vi "missing_Peak2.vi"(8 "Width":dbl=0.02 format="%#_13g", 9 "Average Spacing":dbl=1.0 format="%#_13g") -> (0 "Missing Peaks":i32[](array[numeric])=[3, 4, 7, 8, 9], 3 "Padded Peak Locations":i32[](array[numeric])=[1, 2, 3, 4, 5, 6, 7, 8, 9, 10])   [LabVIEW 2016]
panel:
  in  "array":i32[](array[numeric])
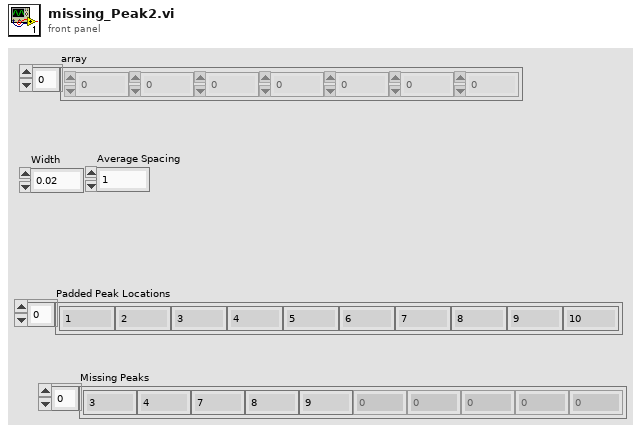
[diagram p1: front panel]
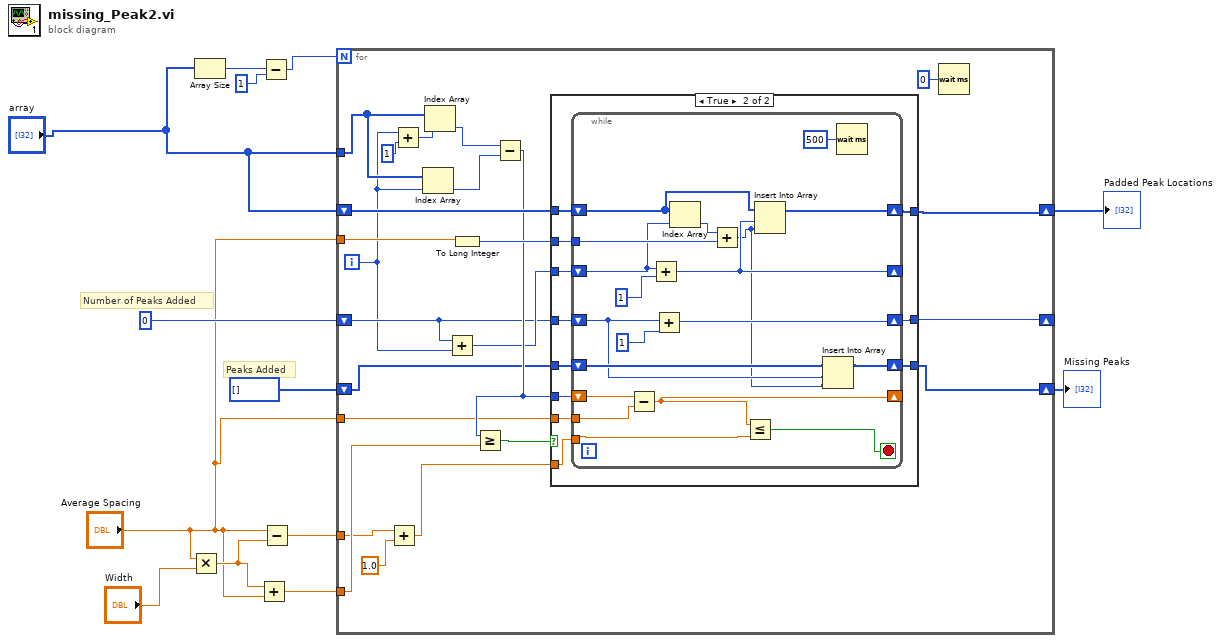
[diagram p0: block diagram]
diagram:
  # "Peaks Added"
  # "Number of Peaks Added"
  n1 = Multiply(x="Average Spacing", y="Width") -> (x*y=w10:dbl)
  n2 = Array Size(array="array") -> (size(s)=w13:i32)
  n3 = Add(x=w10, y="Average Spacing") -> (x+y=w7:dbl)
  n4 = Subtract(x=w13, y=1) -> (x-y=w11:i32)
  n5 = Subtract(x="Average Spacing", y=w10) -> (x-y=w8:dbl)
  n6 = for {
    N: w11 -> [_]
    tunnel: "array" -> [w31]
    tunnel: w8 -> [w19]
    tunnel: w7 -> [w25]
    shift-right: [w29] -> w6
    shift-left: "array" -> [w30]
    tunnel: "Average Spacing" -> [w24]
    shift-right: [w22] -> _
    shift-left: 0 -> [w21]
    shift-right: [w15] -> w3
    shift-left: i32[] [] ("array") -> [w16]
    tunnel: "Average Spacing" -> [w14]
    i -> [w20]
    n7 = Add(x=w19, y=1.0) -> (x+y=w17:dbl)
    n8 = Add(x=w20, y=1) -> (x+y=w36:i32)
    n9 = Index Array(array=w31, index=w20) -> (element=w33:i32)
    n10 = Index Array(array=w31, index=w36) -> (element=w34:i32)
    n11 = Add(x=w21, y=w20) -> (x+y=w23:i32)
    n12 = To Long Integer(number=w24) -> (32bit integer=w28:i32)
    n13 = Subtract(x=w34, y=w33) -> (x-y=w26:i32)
    n14 = Greater Or Equal?(x=w26, y=w25) -> (x >= y?=w32:bool)
    n15 = case shown="True" w32 {
      tunnel: w30 -> [w39 w49]
      tunnel: w26 -> [_ w50]
      tunnel: w23 -> [_ w48]
      tunnel: w28 -> [_ w47]
      tunnel: [w39 w46] -> w29
      tunnel: w21 -> [w38 w45]
      tunnel: [w38 w44] -> w22
      tunnel: w17 -> [_ w43]
      tunnel: w16 -> [w37 w42]
      tunnel: [w37 w41] -> w15
      tunnel: w14 -> [_ w40]
      frame False {
      }
      frame True {
        n16 = while {
          shift-right: [w67] -> _
          shift-left: w50 -> [w69]
          shift-right: [w65] -> w46
          shift-left: w49 -> [w64]
          shift-right: [w60] -> _
          shift-left: w48 -> [w62]
          tunnel: w47 -> [w63]
          shift-right: [w57] -> w44
          shift-left: w45 -> [w53]
          tunnel: w43 -> [w56]
          shift-right: [w55] -> w41
          shift-left: w42 -> [w54]
          tunnel: w40 -> [w51]
          stop <- w68 stop-if-true
          n17 = Subtract(x=w69, y=w51) -> (x-y=w67:dbl)
          n18 = Add(x=w62, y=1) -> (x+y=w60:i32)
          n19 = Add(x=w53, y=1) -> (x+y=w57:i32)
          n20 = Index Array(array=w64, index=w62) -> (element=w59:i32)
          n21 = Add(x=w59, y=w63) -> (x+y=w52:i32)
          n22 = Less Or Equal?(x=w67, y=w56) -> (x <= y?=w68:bool)
          n23 = Insert Into Array(array=w64, index=w60, new element=w52) -> (w65:i32[])
          n24 = Insert Into Array(array=w54, index=w53, new element=w52) -> (w55:i32[])
          n25 = Wait (ms)(milliseconds to wait=u32 500) -> ()  [unwired: 1 out]
        }
      }
    }
    n26 = Wait (ms)(milliseconds to wait=u32 0) -> ()  [unwired: 1 out]
  }
  "Padded Peak Locations" <- w6
  "Missing Peaks" <- w3
